vi "Handle Local Error.vi"(8 "error in":errorcluster) -> (0 "error out":errorcluster)   [LabVIEW 2017, in "Error Handler.lvlib"]
uses:
  Error Handler.lvlib
  User Events/TypeDefs/Shutdown UE FGV Command.ctl
  <vilib>/Utility/error.llb/DialogType.ctl
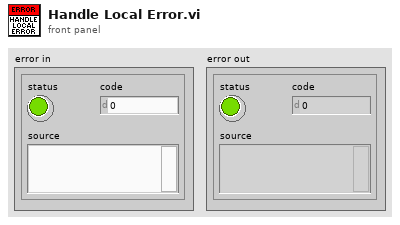
[diagram p1: front panel]
types:
  T1 = enum16{"open", "replace", "create", "open or create", "replace or create", "replace or create with confirmation"}
  T2 = typedef "Shutdown UE FGV Command.ctl" = enum16{"create", "get", "destroy"}
  T3 = typedef "DialogType.ctl" = u16
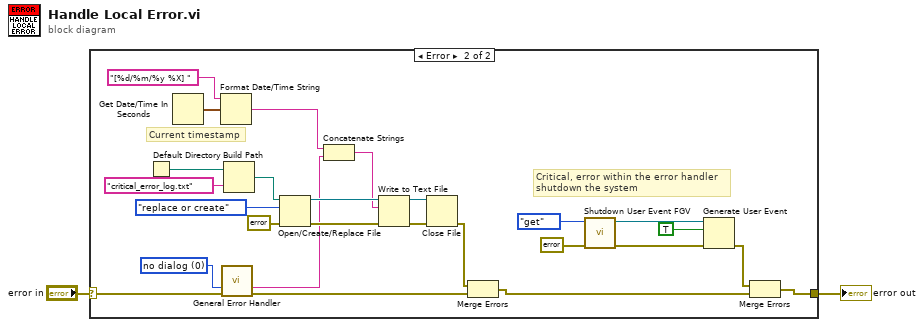
[diagram p0: block diagram]
diagram:
  n1 = case shown="Error" "error in" {
    selector: "error in" -> [w3 w15]
    tunnel: [w3 w23] -> w1
    frame No Error {
    }
    frame Error {
      w14 = T3 0 items=["no dialog", "OK message", "continue or stop message", "OK message + warnings", "continue/stop + warnings"] ("type of dialog (OK msg:1)")
      # "Current timestamp"
      # "Critical, error within the error handler\nshutdown the system"
      n2 = Default Directory() -> (w21:path)
      n3 = Get Date/Time In Seconds() -> (seconds since 1Jan1904=w13:timestamp)
      n4 = Format Date/Time String(time format string (%c)="[%d/%m/%y %X] ", seconds (now)=w13) -> (date/time string=w11:string)  [unwired: 1 in]
      n5 = call <vilib>:"General Error Handler.vi"("type of dialog (OK msg:1)"=w14, "error in (no error)"=w15) -> ("message"=w10:string, "error out"=w5:errorcluster)  [unwired: 9 in, 3 out]
      n6 = Build Path(base path=w21, name or relative path="critical_error_log.txt") -> (appended path=w19:path)
      n7 = Open/Create/Replace File(file path (use dialog)=w19, error in=errorcluster {"status"=FALSE, "code"=0, "source"=""}, operation (0:open)=T1."replace or create") -> (refnum out=w16:refnum<file>, error out=w17:errorcluster)  [unwired: 3 in, 1 out]
      n8 = Concatenate Strings(w11, w10) -> (w9:string)
      n9 = Write to Text File(file (use dialog)=w16, text=w9, error in=w17) -> (refnum out=w7:refnum<file>, error out=w8:errorcluster)  [unwired: 1 in, 1 out]
      n10 = Close File(refnum=w7, error in=w8) -> (error out=w6:errorcluster)  [unwired: 1 out]
      n11 = Merge Errors(w6, w5) -> (w4:errorcluster)
      n12 = call "Shutdown User Event FGV.vi"("error in"=errorcluster {"status"=FALSE, "code"=0, "source"=""}, "command"=Shutdown_UE_FGV_Command."get" ("Command")) -> ("error out"=w27:errorcluster, "shutdown user event"=w26:refnum<user-event>)  [unwired: 8 in]
      n13 = Generate User Event(user event=w26, event data cluster=TRUE ("event data"), error in=w27) -> (error out=w24:errorcluster)  [unwired: 1 in, 1 out]
      n14 = Merge Errors(w24, w4) -> (w23:errorcluster)
    }
  }
  "error out" <- w1
